vi "Log_CreateFolder.vi"(8 "error in (no error)":errorcluster) -> (0 "error out":errorcluster, 3 "created path":path)   [LabVIEW 2013]
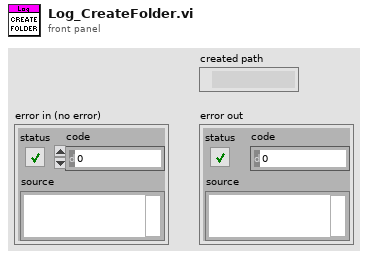
[diagram p1: front panel]
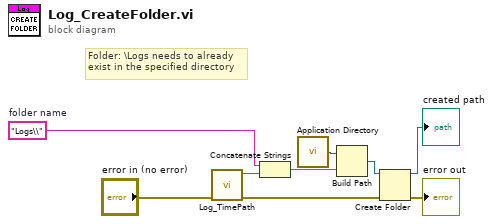
[diagram p0: block diagram]
diagram:
  w1 = "Logs\\"  # folder name
  # "Folder: \\Logs needs to already\nexist in the specified directory"
  n1 = call "Log_TimePath.vi"("error in (no error)"="error in (no error)") -> ("error out"=w3:errorcluster, "result string"=w2:string)  [unwired: 9 in]
  n2 = Concatenate Strings(w1, w2) -> (w7:string)
  n3 = call <vilib>:"Application Directory.vi"() -> ("Application Directory"=w6:path)
  n4 = Build Path(base path=w6, name or relative path=w7) -> (appended path=w8:path)
  n5 = Create Folder(path (use dialog)=w8, error in=w3) -> (created path=→"created path":path, error out=→"error out":errorcluster)  [unwired: 1 in, 1 out]
